vi "Main.vi"() -> ()   [LabVIEW 2014, in "mySynthesizer.lvlib"]
uses:
  mySynthesizer.lvlib
panel:
  out "error in (no error) 2":errorcluster
  in  "error in (no error)":errorcluster
  in  "stop":bool
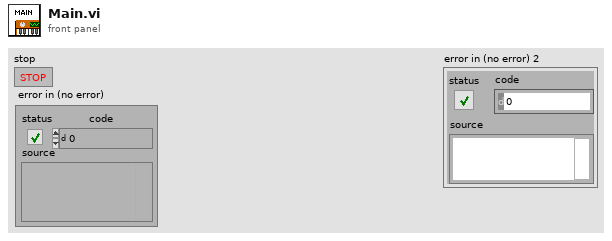
[diagram p1: front panel]
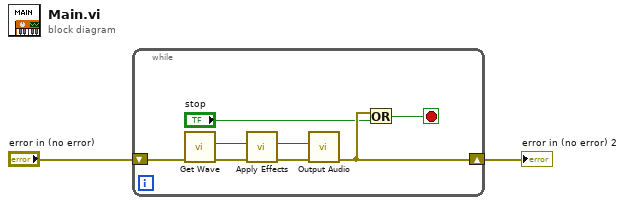
[diagram p0: block diagram]
diagram:
  n1 = while {
    shift-right: [w5] -> w1
    shift-left: "error in (no error)" -> [w6]
    stop <- w4 stop-if-true
    n2 = call "Get Wave.vi"("error in (no error)"=w6) -> ("error out"=w9:errorcluster, "Instrument Level Processing out"=w10:variant)  [unwired: 9 in]
    n3 = call "Apply Effects.vi"("error in (no error)"=w9, "Instrument In"=w10) -> ("error out"=w7:errorcluster, "Instrument out"=w8:variant)  [unwired: 8 in]
    n4 = call "Output Audio.vi"("error in (no error)"=w7, "Instrument In"=w8) -> ("error out"=w5:errorcluster)  [unwired: 8 in, 1 out]
    n5 = Or(x=w5, y="stop") -> (x .or. y?=w4:bool)
  }
  "error in (no error) 2" <- w1
